vi "Index of Object.vi"(8 "error in (no error)":errorcluster caption="错误输入（无错误）", 9 "startIndex":i32, 10 "anything":variant caption="任何数据", 11 "ArrayListClass 输入":refnum<class "ArrayListClass.lvclass"> caption="DNL_LabVIEW Object in") -> (0 "error out":errorcluster caption="错误输出", 1 "IndexOf":i32, 3 "ArrayListClass 输出":refnum<class "ArrayListClass.lvclass"> caption="DNL_LabVIEW Object out")   [LabVIEW 2012, in "ArrayListClass.lvclass"]
uses:
  ArrayListClass.lvclass
  ArrayListClass.lvclass/ArrayListClass.ctl
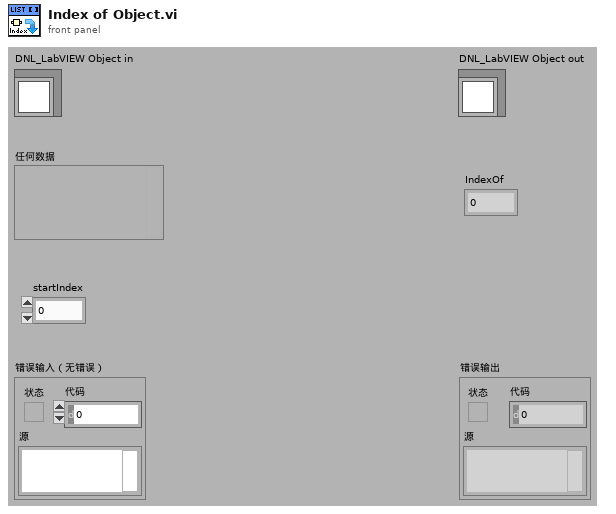
[diagram p1: front panel]
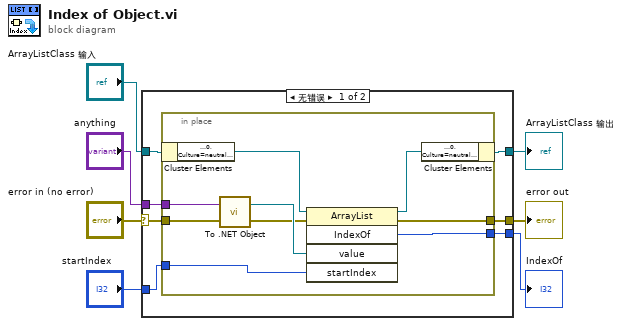
[diagram p0: block diagram]
diagram:
  n1 = case shown="无错误" "error in (no error)" {
    selector: "error in (no error)" -> [w11 w25]
    tunnel: [w10 w25] -> w6
    tunnel: [w12 w24] -> w4
    tunnel: "ArrayListClass 输入" -> [w14 w24]
    tunnel: "anything" -> [w13 _]
    tunnel: "startIndex" -> [w9 _]
    tunnel: [w8 _] -> w1
    frame No Error {
      n2 = in-place {
        in-place-border: w13 -> [w20]
        in-place-border: w11 -> [w18]
        in-place-border: [w19] -> w10
        in-place-border: w9 -> [w16]
        in-place-border: [w15] -> w8
        n3 = in-place-cluster #1(w14) -> ("ArrayList"=w23:refnum<k24>)
        n4 = call <vilib>:"To .NET Object.vi"("error in (no error)"=w18, "anything"=w20) -> ("error out"=w17:errorcluster, ".NET object"=w21:refnum<k24>)
        n5 = invoke class="ArrayList" method="IndexOf"(reference=w23, error in=w17, "value"=w21, "startIndex"=w16) -> (reference out=w22:refnum<k24>, error out=w19:errorcluster, "IndexOf"=w15:i32)  [unwired: 1 in, 2 out]
        n6 = in-place-cluster #1("ArrayList"=w22) -> (w12:refnum<class "ArrayListClass.lvclass">)
      }
    }
    frame Error {
    }
  }
  "error out" <- w6
  "ArrayListClass 输出" <- w4
  "IndexOf" <- w1
